vi "LakeShore218_02_Main.vi"() -> ()   [LabVIEW 2019]
uses:
  LakeShore218_Global.vi
panel:
  out "T_Cernox":dbl caption="Ch 7: Cernox" format="%.2f"
  out "status_rec":bool=TRUE caption="Logging Status"
  out "Last Measured":timestamp format="%<%Y-%m-%d %H:%M:%S>T"
  out "Chart":waveform(dbl)[](graph)=[{"t0"=timestamp(3753816869.352795 s since 1904-01-01), "dt"=1.0, "Y"=[-2.5246], "attributes"=variant("NI_ChannelName"=variant(string "Target Top Up"))}, {"t0"=timestamp(3753816869.352795 s since 1904-01-01), "dt"=1.0, "Y"=[-2.5246], "attributes"=variant("NI_ChannelName"=variant(string "Target Top Center"))}, {"t0"=timestamp(3753816869.352795 s since 1904-01-01), "dt"=1.0, "Y"=[-2.5246], "attributes"=variant("NI_ChannelName"=variant(string "Target Top Down"))}, {"t0"=timestamp(3753816869.352795 s since 1904-01-01), "dt"=1.0, "Y"=[-2.5246], "attributes"=variant("NI_ChannelName"=variant(string "Target Bottom Up"))}, {"t0"=timestamp(3753816869.352795 s since 1904-01-01), "dt"=1.0, "Y"=[2.5246], "attributes"=variant("NI_ChannelName"=variant(string "Target Bottom Center"))}, {"t0"=timestamp(3753816869.352795 s since 1904-01-01), "dt"=1.0, "Y"=[2.5246], "attributes"=variant("NI_ChannelName"=variant(string "Target Bottom Down"))}, {"t0"=timestamp(3753816869.352795 s since 1904-01-01), "dt"=1.0, "Y"=[2.5246], "attributes"=variant("NI_ChannelName"=variant(string "Target Cernox"))}, {"t0"=timestamp(3753816869.352795 s since 1904-01-01), "dt"=1.0, "Y"=[2.5246], "attributes"=variant("NI_ChannelName"=variant(string "n/a"))}]
  in  "Interval":u32=1000
  out "status":bool=TRUE
  out "value_array":dbl[](array[numeric]) caption="Last Readings" format="%.1f"
  in  "stop":bool
  in  "VISA":refnum<visa-resource-name>="GPIB0::3::INSTR"
  # "LakeShore218 #02: Target Cup Temperature"
  # "ms"
  # "W"
  # "K"
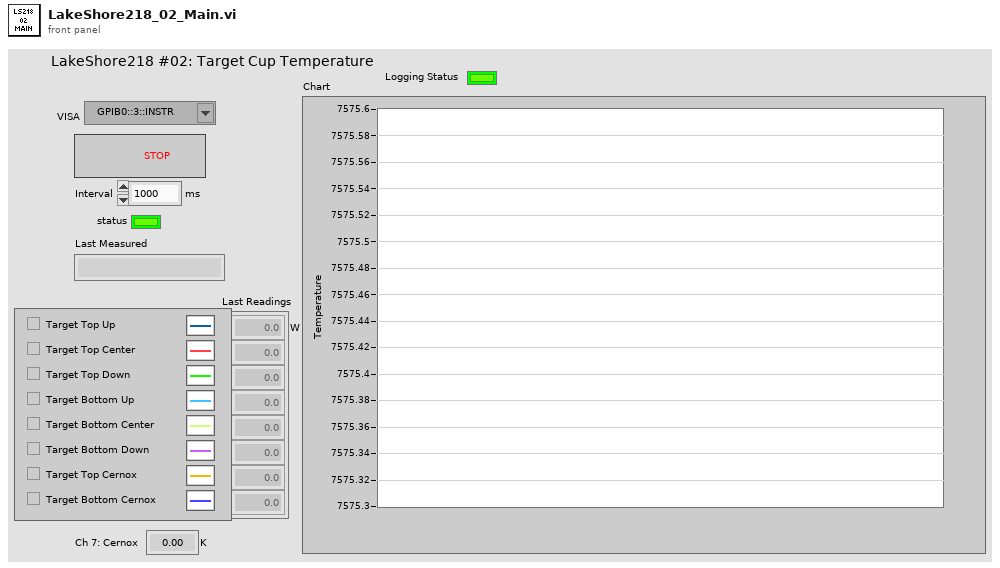
[diagram p1: front panel]
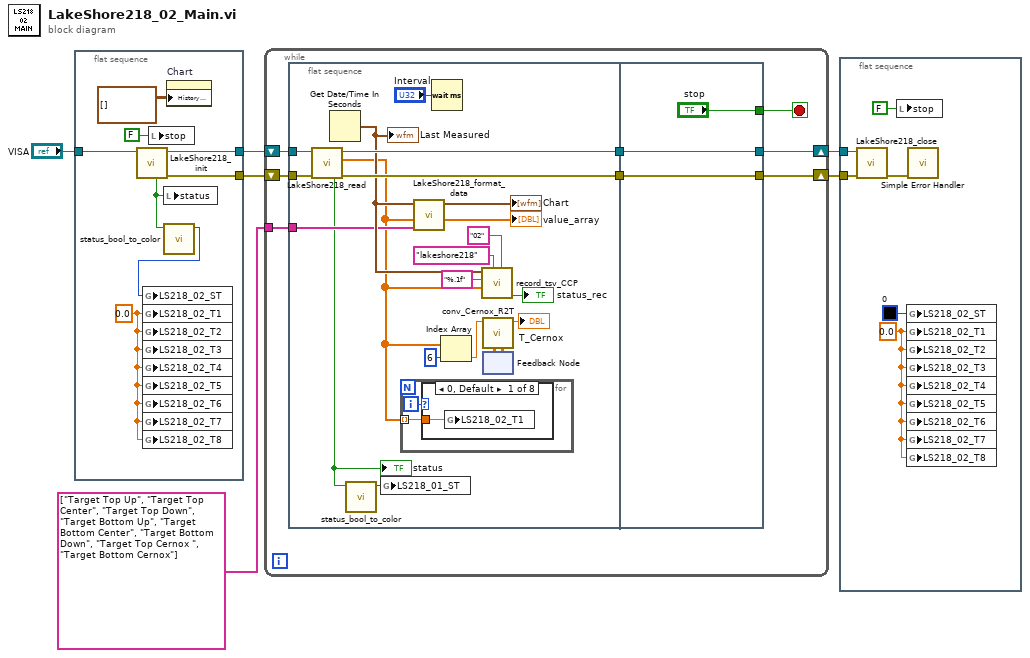
[diagram p0: block diagram]
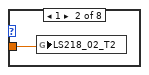
[diagram p2: hidden frame]
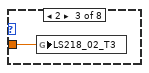
[diagram p3: hidden frame]
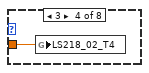
[diagram p4: hidden frame]
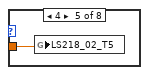
[diagram p5: hidden frame]
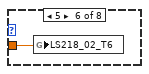
[diagram p6: hidden frame]
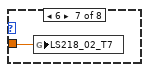
[diagram p7: hidden frame]
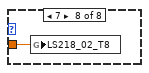
[diagram p8: hidden frame]
diagram:
  n1 = flat-sequence {
    tunnel: [w14] -> w6
    tunnel: [w13] -> w5
    tunnel: "VISA" -> [w12]
    frame #0 {
      w9 = 0.0 ("LS218_01_T1")
      n2 = call "LakeShore218_init.vi"("VISA in"=w12) -> ("error out"=w14:errorcluster, "VISA out"=w13:refnum<visa-resource-name>, "status"=w8:bool)  [unwired: 8 in]
      n3 = global write "LakeShore218_Global.vi" "LS218_02_T1"(w9) -> ()
      n4 = global write "LakeShore218_Global.vi" "LS218_02_T2"(w9) -> ()
      n5 = global write "LakeShore218_Global.vi" "LS218_02_T3"(w9) -> ()
      n6 = global write "LakeShore218_Global.vi" "LS218_02_T4"(w9) -> ()
      n7 = global write "LakeShore218_Global.vi" "LS218_02_T5"(w9) -> ()
      n8 = global write "LakeShore218_Global.vi" "LS218_02_T6"(w9) -> ()
      n9 = global write "LakeShore218_Global.vi" "LS218_02_T7"(w9) -> ()
      n10 = global write "LakeShore218_Global.vi" "LS218_02_T8"(w9) -> ()
      n11 = local write "stop"(FALSE ("stop")) -> ()
      n12 = local write "status"(w8) -> ()
      n13 = call "status_bool_to_color.vi"("status_bool_1"=w8) -> ("status_color"=w7:u32)  [unwired: 10 in]
      n14 = global write "LakeShore218_Global.vi" "LS218_02_ST"(w7) -> ()
      n15 = property on="Chart" class="WFChart (strict)"("History Data"=waveform(dbl)[][] []) -> ()  [unwired: 2 in, 2 out]
    }
  }
  n16 = while {
    shift-right: [w20] -> w3
    shift-left: w5 -> [w21]
    shift-right: [w19] -> w2
    shift-left: w6 -> [w22]
    tunnel: string[] ["Target Top Up", "Target Top Center", "Target Top Down", "Target Bottom Up", "Target Bottom Center", "Target Bottom Down", "Target Top Cernox ", "Target Bottom Cernox"] ("format_array") -> [w15]
    stop <- w16 stop-if-true
    n17 = flat-sequence {
      tunnel: w22 -> [w43]
      tunnel: w21 -> [w42]
      tunnel: [w40] -> w18
      tunnel: [w39] -> w17
      tunnel: w15 -> [w32]
      tunnel: [w55] -> w19
      tunnel: [w56] -> w20
      tunnel: w18 -> [w56]
      tunnel: w17 -> [w55]
      tunnel: ["stop"] -> w16
      frame #0 {
        n18 = call "LakeShore218_read.vi"("error in"=w43, "VISA in"=w42) -> ("error out"=w39:errorcluster, "value_array"=w23:dbl[], "VISA out"=w40:refnum<visa-resource-name>, "status"=w24:bool)  [unwired: 6 in]
        "status" <- w24
        n19 = Get Date/Time In Seconds() -> (seconds since 1Jan1904=w36:timestamp)
        "Last Measured" <- w36
        n20 = call "status_bool_to_color.vi"("status_bool_1"=w24) -> ("status_color"=w25:u32)  [unwired: 10 in]
        n21 = global write "LakeShore218_Global.vi" "LS218_01_ST"(w25) -> ()
        n22 = for {
          tunnel: w23 -> [w44] mode=indexing
          i -> [w45]
          n23 = case shown="0, Default" w45 {
            tunnel: w44 -> [w46 w47 w48 w49 w50 w51 w52 w53]
            frame 0, Default {
              n24 = global write "LakeShore218_Global.vi" "LS218_02_T1"(w46) -> ()
            }
            frame 1 {
              n25 = global write "LakeShore218_Global.vi" "LS218_02_T2"(w47) -> ()
            }
            frame 2 {
              n26 = global write "LakeShore218_Global.vi" "LS218_02_T3"(w48) -> ()
            }
            frame 3 {
              n27 = global write "LakeShore218_Global.vi" "LS218_02_T4"(w49) -> ()
            }
            frame 4 {
              n28 = global write "LakeShore218_Global.vi" "LS218_02_T5"(w50) -> ()
            }
            frame 5 {
              n29 = global write "LakeShore218_Global.vi" "LS218_02_T6"(w51) -> ()
            }
            frame 6 {
              n30 = global write "LakeShore218_Global.vi" "LS218_02_T7"(w52) -> ()
            }
            frame 7 {
              n31 = global write "LakeShore218_Global.vi" "LS218_02_T8"(w53) -> ()
            }
          }
        }
        n32 = call "LakeShore218_format_data.vi"("name_array"=w32, "value_array"=w23, "time"=w36) -> ("value_array_out"=→"value_array":dbl[], "waveform_array"=→"Chart":waveform(dbl)[])  [unwired: 7 in]
        n33 = Wait (ms)(milliseconds to wait="Interval") -> ()  [unwired: 1 out]
        n34 = Index Array(array=w23, index=6) -> (element=w27:dbl)
        n35 = call "record_tsv_CCP.vi"("file_name"="02", "folder_name"="lakeshore218", "value_array"=w23, "format"="%.1f", "time"=w36) -> ("status"=→"status_rec":bool)  [unwired: 5 in, 1 out]
        n36 = feedback #1() -> (w28:dbl[][])  [unwired: 1 in]
        n37 = call "conv_Cernox_R2T.vi"("data_in"=w28, "R"=w27) -> ("T"=→"T_Cernox":dbl, "data_out"=w29:dbl[][])  [unwired: 7 in, 1 out]
        n38 = feedback-in #1(w29) -> ()
      }
      frame #1 {
      }
    }
  }
  n39 = flat-sequence {
    tunnel: w3 -> [w62]
    tunnel: w2 -> [w61]
    frame #0 {
      w58 = 0.0 ("LS218_01_T1")
      n40 = call "LakeShore218_close.vi"("error in"=w61, "VISA in"=w62) -> ("error out"=w60:errorcluster)  [unwired: 9 in]
      n41 = local write "stop"(FALSE ("stop")) -> ()
      n42 = global write "LakeShore218_Global.vi" "LS218_02_ST"(u32 0 ("LS218_02_ST")) -> ()
      n43 = global write "LakeShore218_Global.vi" "LS218_02_T1"(w58) -> ()
      n44 = global write "LakeShore218_Global.vi" "LS218_02_T2"(w58) -> ()
      n45 = global write "LakeShore218_Global.vi" "LS218_02_T3"(w58) -> ()
      n46 = global write "LakeShore218_Global.vi" "LS218_02_T4"(w58) -> ()
      n47 = global write "LakeShore218_Global.vi" "LS218_02_T5"(w58) -> ()
      n48 = global write "LakeShore218_Global.vi" "LS218_02_T6"(w58) -> ()
      n49 = global write "LakeShore218_Global.vi" "LS218_02_T7"(w58) -> ()
      n50 = global write "LakeShore218_Global.vi" "LS218_02_T8"(w58) -> ()
      n51 = call <vilib>:"Simple Error Handler.vi"("error in (no error)"=w60) -> ()  [unwired: 4 in, 5 out]
    }
  }
